vi "LuaPush.vi"(1 "Variant":variant, 2 "L In":u64, 3 "Lua Dll":path) -> (0 "L Out":u64)   [LabVIEW 2014]
uses:
  <vilib>/Utility/VariantDataType/Type.ctl
  <vilib>/Utility/VariantDataType/VariantType.lvlib
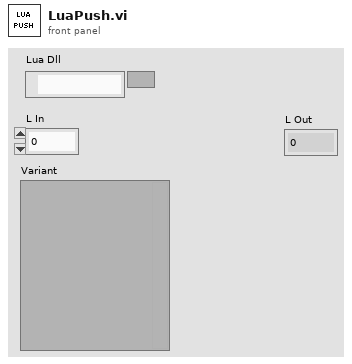
[diagram p1: front panel]
types:
  T1 = typedef "VariantType.lvlib/Type.ctl" = enum8{"Invalid Type", "Void", "I8", "I16", "I32", "I64", "U8", "U16", "U32", "U64", "Single Float", "Double Float", "Extended Float", "Single Complex", "Double Complex", "Extended Complex", "Enum U8", "Enum U16", "Enum U32", "Enum U64", "Single Float With Unit", "Double Float With Unit", "Extended Float With Unit", "Single Complex with Unit", "Double Complex with Unit", "Extended Complex with Unit", "Boolean", "String", "Path", "Picture", "Tag", "Array", "Cluster", "Variant", "LV Variant", "Waveform", "Timestamp", "Digital Waveform", "Digital Data", "ExpressData", "Refnum", "External Data", "VI", "Poly VI", "LabVIEW Class Instance", "Fixed Point"}
  T2 = typedef "VariantType.lvlib/RefnumType.ctl" = enum16{"NotARefnum", "UnknownRefnum", "Generic", "Datalog", "ByteStream", "Device", "Occurence", "TCPNetConnection", "Auto", "Menu", "Imaq", "Hardware", "DataSocket", "Visa", "IVI", "UDPNetConnection", "Notifier", "Queue", "Irda", "EventReg", "DotNet", "UserEvent", "Callback", "UNUSED_EMPTY_POSITION", "BlueToothNetConnection", "LVObjApp", "LVObjVI", "LVObjUnknown", "GenericClass", "UserDefinedRefnumTag", "DataValue", "RT FIFO", "TDMS File"}
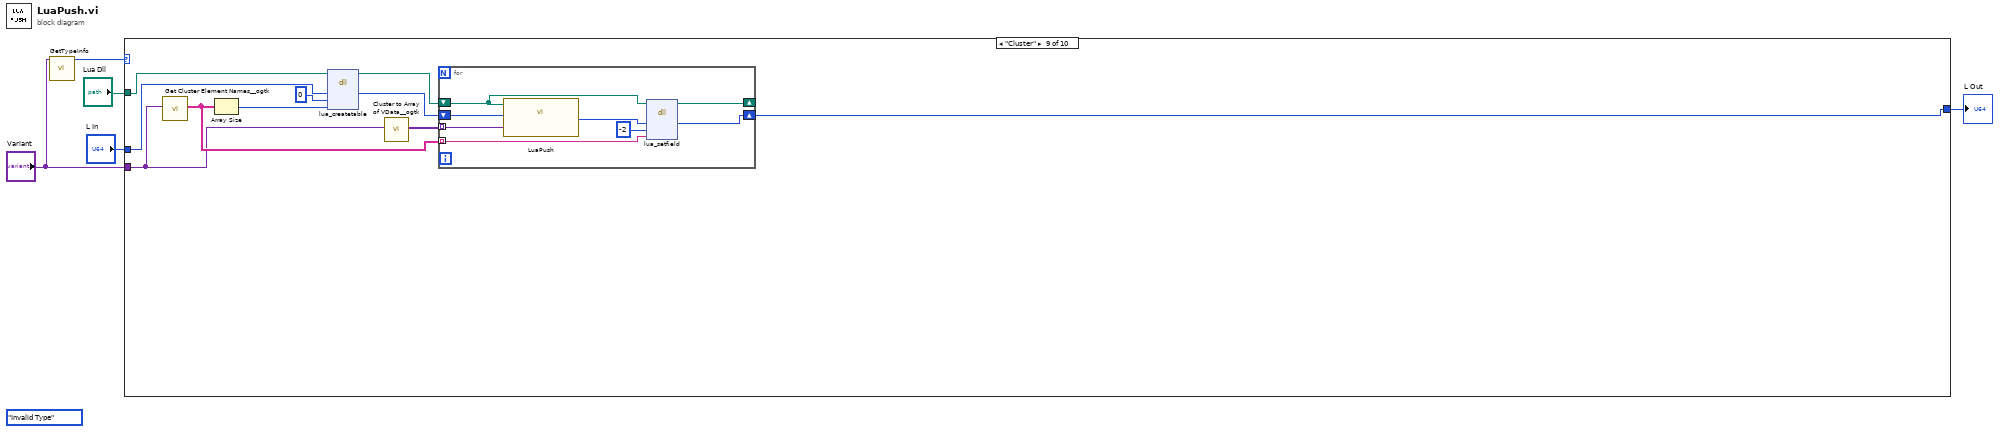
[diagram p0: block diagram]
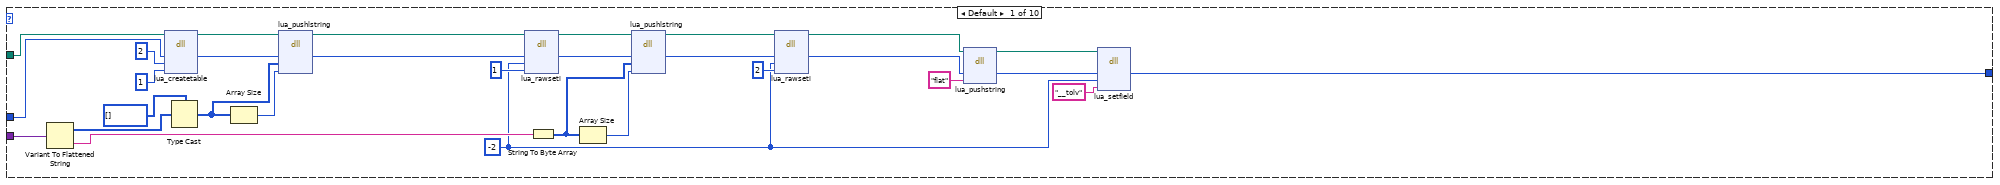
[diagram p2: hidden frame]
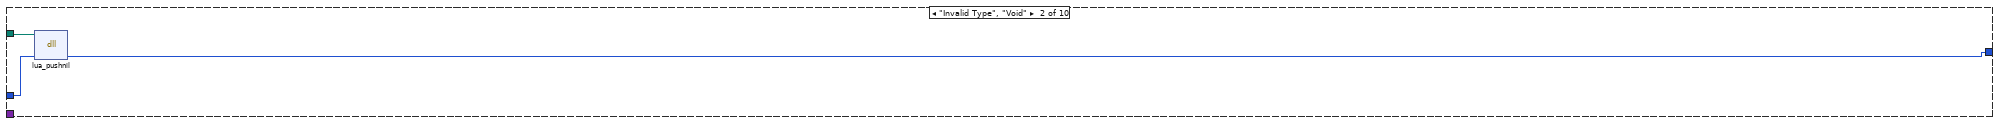
[diagram p3: hidden frame]
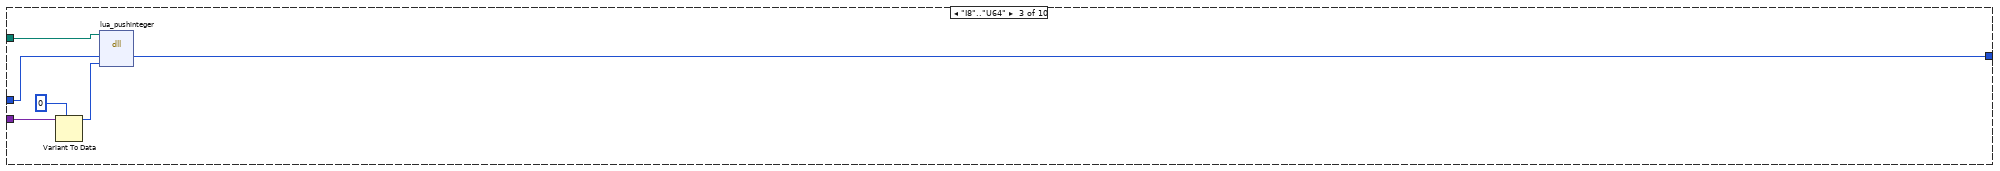
[diagram p4: hidden frame]
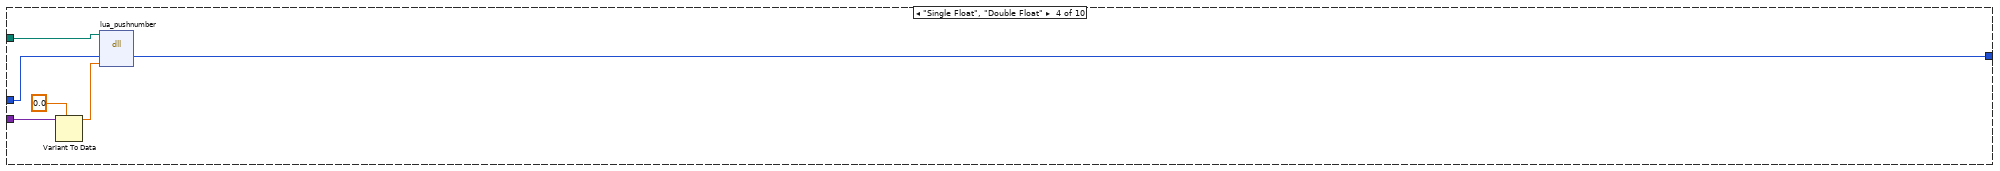
[diagram p5: hidden frame]
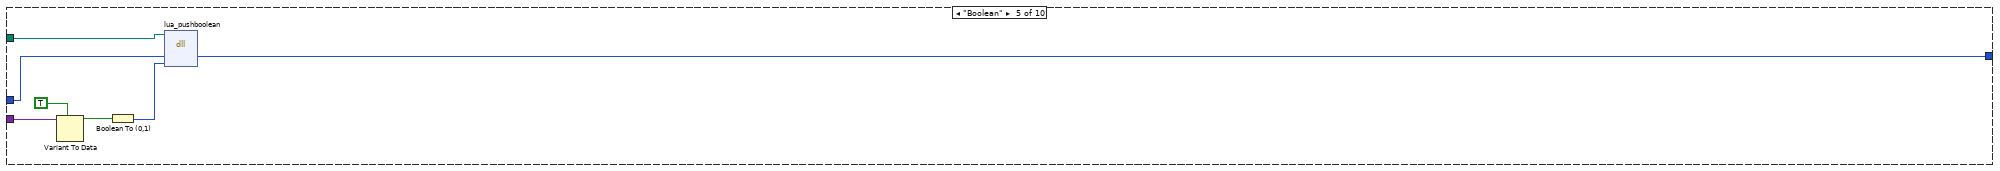
[diagram p6: hidden frame]
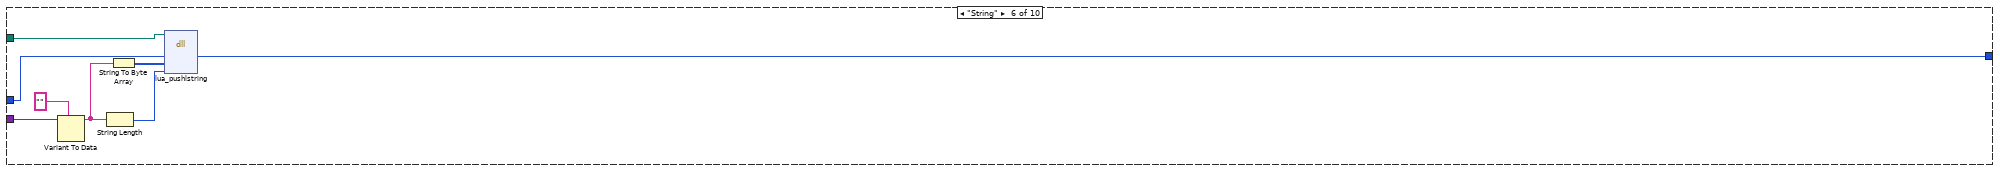
[diagram p7: hidden frame]
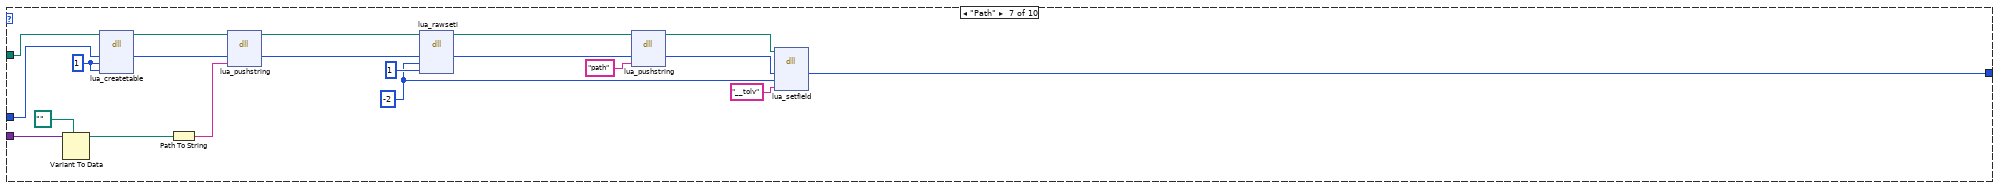
[diagram p8: hidden frame]
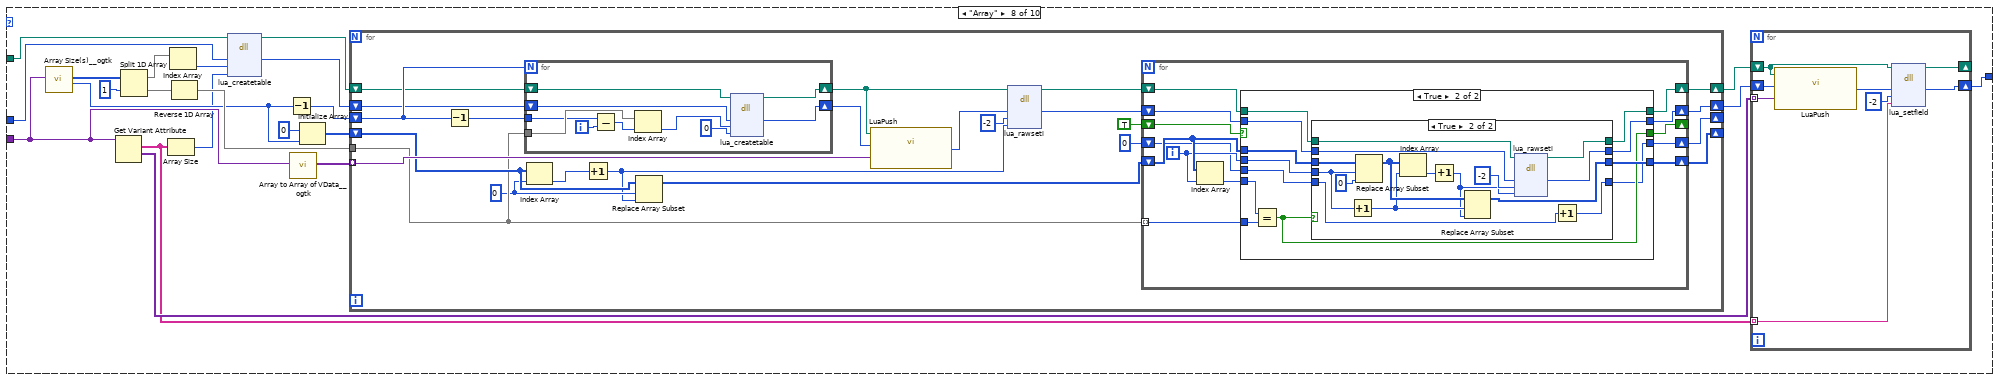
[diagram p9: hidden frame]
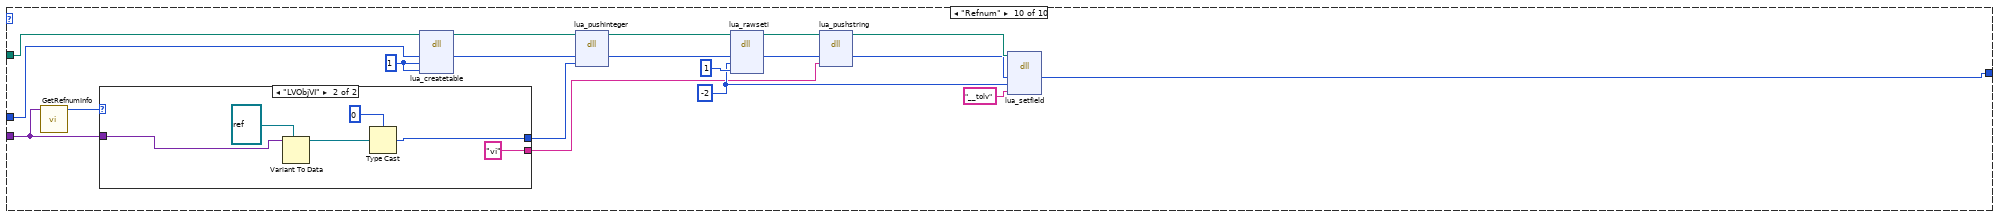
[diagram p12: hidden frame]
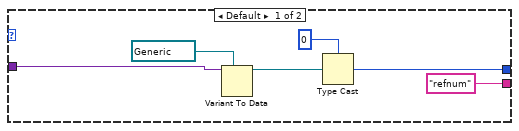
[diagram p13: hidden frame]
diagram:
  (unwired) Type."Invalid Type" ("Type Enum")
  n1 = call <vilib>:"GetTypeInfo.vi"("Variant"="Variant") -> ("Type Enum"=w5:T1)  [unwired: 6 in, 4 out]
  n2 = case shown="\"Cluster\"" w5 {
    tunnel: "Lua Dll" -> [w35 w38 w41 w47 w56 w64 w77 w95 w206 w221]
    tunnel: "L In" -> [w34 w37 w40 w46 w55 w63 w76 w93 w207 w219]
    tunnel: "Variant" -> [w26 _ w44 w50 w57 w65 w71 w99 w199 w223]
    tunnel: [w6 w36 w39 w45 w51 w58 w66 w86 w201 w216] -> w1
    frame Default {
      w7 = -2 ("n")
      n3 = Variant To Flattened String(Variant=w26) -> (data string=w19:string, 1:w25:i16[])
      n4 = dll-call lib="lua5.dll" fn="lua_createtable"(path in=w35, "L"=w34, "narr"=2, "nrec"=1) -> (path out=w22:path, "L"=w23:u64)  [unwired: 5 in, 1 out]
      n5 = Type Cast(type=u8[] [], x=w25) -> (*(type *) &x=w10:u8[])
      n6 = Array Size(array=w10) -> (size(s)=w9:i32)
      n7 = dll-call lib="lua5.dll" fn="lua_pushlstring"(path in=w22, "L"=w23, "str"=w10, "len"=w9) -> (path out=w21:path, "L"=w20:u64)  [unwired: 5 in, 1 out]
      n8 = dll-call lib="lua5.dll" fn="lua_rawseti"(path in=w21, "L"=w20, "n"=w7, "i"=1) -> (path out=w18:path, "L"=w15:u64)  [unwired: 5 in, 1 out]
      n9 = String To Byte Array(string=w19) -> (unsigned byte array=w12:u8[])
      n10 = Array Size(array=w12) -> (size(s)=w11:i32)
      n11 = dll-call lib="lua5.dll" fn="lua_pushlstring"(path in=w18, "L"=w15, "str"=w12, "len"=w11) -> (path out=w17:path, "L"=w14:u64)  [unwired: 5 in, 1 out]
      n12 = dll-call lib="lua5.dll" fn="lua_rawseti"(path in=w17, "L"=w14, "n"=w7, "i"=2) -> (path out=w16:path, "L"=w13:u64)  [unwired: 5 in, 1 out]
      n13 = dll-call lib="lua5.dll" fn="lua_pushstring"(path in=w16, "L"=w13, "str"="flat") -> (path out=w31:path, "L"=w30:u64)  [unwired: 4 in, 1 out]
      n14 = dll-call lib="lua5.dll" fn="lua_setfield"(path in=w31, "L"=w30, "n"=w7, "i"="__tolv") -> ("L"=w6:u64)  [unwired: 5 in, 2 out]
    }
    frame "Invalid Type", "Void" {
      n15 = dll-call lib="lua5.dll" fn="lua_pushnil"(path in=w38, "L"=w37) -> ("L"=w36:u64)  [unwired: 3 in, 2 out]
    }
    frame "I8".."U64" {
      n16 = Variant To Data(type=i64 0 ("n"), Variant=w44) -> (data=w42:i64)  [unwired: 1 in, 1 out]
      n17 = dll-call lib="lua5.dll" fn="lua_pushinteger"(path in=w41, "L"=w40, "n"=w42) -> ("L"=w39:u64)  [unwired: 4 in, 2 out]
    }
    frame "Single Float", "Double Float" {
      n18 = Variant To Data(type=0.0 ("n"), Variant=w50) -> (data=w48:dbl)  [unwired: 1 in, 1 out]
      n19 = dll-call lib="lua5.dll" fn="lua_pushnumber"(path in=w47, "L"=w46, "n"=w48) -> ("L"=w45:u64)  [unwired: 4 in, 2 out]
    }
    frame "Boolean" {
      n20 = Variant To Data(type=TRUE, Variant=w57) -> (data=w53:bool)  [unwired: 1 in, 1 out]
      n21 = Boolean To (0,1)(Boolean=w53) -> (0, 1=w52:i16)
      n22 = dll-call lib="lua5.dll" fn="lua_pushboolean"(path in=w56, "L"=w55, "n"=w52) -> ("L"=w51:u64)  [unwired: 4 in, 2 out]
    }
    frame "String" {
      n23 = Variant To Data(type="", Variant=w65) -> (data=w60:string)  [unwired: 1 in, 1 out]
      n24 = String Length(string=w60) -> (length=w61:i32)
      n25 = String To Byte Array(string=w60) -> (unsigned byte array=w59:u8[])
      n26 = dll-call lib="lua5.dll" fn="lua_pushlstring"(path in=w64, "L"=w63, "str"=w59, "len"=w61) -> ("L"=w58:u64)  [unwired: 5 in, 2 out]
    }
    frame "Path" {
      w78 = 1 ("narr")
      w79 = -2 ("n")
      n27 = Variant To Data(type=path "" ("path"), Variant=w71) -> (data=w69:path)  [unwired: 1 in, 1 out]
      n28 = dll-call lib="lua5.dll" fn="lua_createtable"(path in=w77, "L"=w76, "narr"=w78, "nrec"=w78) -> (path out=w75:path, "L"=w73:u64)  [unwired: 5 in, 1 out]
      n29 = Path To String(path=w69) -> (string=w68:string)
      n30 = dll-call lib="lua5.dll" fn="lua_pushstring"(path in=w75, "L"=w73, "str"=w68) -> (path out=w74:path, "L"=w72:u64)  [unwired: 4 in, 1 out]
      n31 = dll-call lib="lua5.dll" fn="lua_rawseti"(path in=w74, "L"=w72, "n"=w79, "i"=1) -> (path out=w82:path, "L"=w81:u64)  [unwired: 5 in, 1 out]
      n32 = dll-call lib="lua5.dll" fn="lua_pushstring"(path in=w82, "L"=w81, "str"="path") -> (path out=w85:path, "L"=w84:u64)  [unwired: 4 in, 1 out]
      n33 = dll-call lib="lua5.dll" fn="lua_setfield"(path in=w85, "L"=w84, "n"=w79, "i"="__tolv") -> ("L"=w66:u64)  [unwired: 5 in, 2 out]
    }
    frame "Array" {
      n34 = call <userlib>:"Array Size(s)__ogtk.vi"("Array"=w99) -> ("N dims"=w100:u32, "Size(s)"=w101:u32[])  [unwired: 8 in, 1 out]
      n35 = Get Variant Attribute(Variant=w99) -> (names=w97:string[], values=w98:variant[])  [unwired: 3 in, 2 out]
      n36 = Split 1D Array(array=w101, index=1) -> (first subarray=w88:u32[], second subarray=w103:u32[])
      n37 = Array Size(array=w97) -> (size(s)=w96:i32)
      n38 = Index Array(array=w88) -> (element=w87:u32)  [unwired: 1 in]
      n39 = Reverse 1D Array(array=w103) -> (reversed array=w104:u32[])
      n40 = dll-call lib="lua5.dll" fn="lua_createtable"(path in=w95, "L"=w93, "narr"=w87, "nrec"=w96) -> (path out=w94:path, "L"=w92:u64)  [unwired: 5 in, 1 out]
      n41 = Decrement(x=w100) -> (x-1=w89:u32)
      n42 = call <userlib>:"Array to Array of VData__ogtk.vi"("MultiD Array"=w99) -> ("1D Array of Variants"=w107:variant[])  [unwired: 9 in, 1 out]
      n43 = Initialize Array(0 ("nrec"), w100) -> (w105:i32[])
      n44 = for {
        tunnel: w107 -> [w136] mode=indexing
        shift-right: [w126] -> w91
        shift-left: w94 -> [w122]
        shift-right: [w125] -> w90
        shift-left: w92 -> [w121]
        shift-right: [w129] -> _
        shift-left: w105 -> [w133]
        tunnel: w104 -> [w128]
        shift-right: [w124] -> _
        shift-left: w89 -> [w123]
        w117 = 0 ("index")
        n45 = Decrement(x=w123) -> (x-1=w127:u32)
        n46 = for {
          N: w123 -> [_]
          shift-right: [w139] -> w137
          shift-left: w122 -> [w148]
          shift-right: [w146] -> w120
          shift-left: w121 -> [w147]
          tunnel: w128 -> [w144]
          tunnel: w127 -> [w140]
          i -> [w142]
          n47 = Subtract(x=w140, y=w142) -> (x-y=w141:u32)
          n48 = Index Array(array=w144, index=w141) -> (element=w143:u32)
          n49 = dll-call lib="lua5.dll" fn="lua_createtable"(path in=w148, "L"=w147, "narr"=w143, "nrec"=0) -> (path out=w139:path, "L"=w146:u64)  [unwired: 5 in, 1 out]
        }
        n50 = Index Array(array=w133, index=w117) -> (element=w118:i32)
        n51 = Increment(x=w118) -> (x+1=w116:i32)
        n52 = Replace Array Subset(array=w133, new element=w116, index=w117) -> (w132:i32[])
        n53 = call "LuaPush.vi"("Variant"=w136, "L In"=w120, "Lua Dll"=w137) -> ("L Out"=w135:u64)
        n54 = dll-call lib="lua5.dll" fn="lua_rawseti"(path in=w137, "L"=w135, "n"=-2, "i"=w116) -> (path out=w138:path, "L"=w134:u64)  [unwired: 5 in, 1 out]
        n55 = for {
          shift-right: [w153] -> w129
          shift-left: w132 -> [w157]
          tunnel: w128 -> [w159] mode=indexing
          shift-right: [w151] -> w125
          shift-left: w134 -> [w154]
          shift-right: [w152] -> w126
          shift-left: w138 -> [w155]
          shift-right: [w158] -> _
          shift-left: TRUE -> [w161]
          shift-right: [w149] -> w124
          shift-left: 0 ("new element/subarray") -> [w150]
          i -> [w156]
          n56 = Index Array(array=w157, index=w156) -> (element=w160:i32)
          n57 = case shown="True" w161 {
            selector: w161 -> [w166 _]
            tunnel: [w165 w178] -> w153
            tunnel: [w164 w177] -> w152
            tunnel: [w163 w176] -> w151
            tunnel: w160 -> [_ w175]
            tunnel: w159 -> [_ w174]
            tunnel: [w166 w173] -> w158
            tunnel: w157 -> [w165 w172]
            tunnel: w156 -> [_ w171]
            tunnel: w155 -> [w164 w170]
            tunnel: w154 -> [w163 w169]
            tunnel: w150 -> [w162 w168]
            tunnel: [w162 w167] -> w149
            frame False {
            }
            frame True {
              n58 = Equal?(x=w175, y=w174) -> (x = y?=w173:bool)
              n59 = case shown="True" w173 {
                tunnel: [w180 w189] -> w178
                tunnel: [w182 w194] -> w177
                tunnel: [w181 w193] -> w176
                tunnel: w172 -> [w180 w192]
                tunnel: w171 -> [_ w191]
                tunnel: w170 -> [w182 w186]
                tunnel: w169 -> [w181 w185]
                tunnel: w168 -> [w179 w184]
                tunnel: [w179 w183] -> w167
                frame False {
                }
                frame True {
                  n60 = Increment(x=w191) -> (x+1=w188:i32)
                  n61 = Replace Array Subset(array=w192, new element=0 ("new element/subarray"), index=w191) -> (w190:i32[])
                  n62 = Index Array(array=w190, index=w188) -> (element=w195:i32)
                  n63 = Increment(x=w195) -> (x+1=w187:i32)
                  n64 = Replace Array Subset(array=w190, new element=w187, index=w188) -> (w189:i32[])
                  n65 = dll-call lib="lua5.dll" fn="lua_rawseti"(path in=w186, "L"=w185, "n"=-2, "i"=w187) -> (path out=w194:path, "L"=w193:u64)  [unwired: 5 in, 1 out]
                  n66 = Increment(x=w184) -> (x+1=w183:i32)
                }
              }
            }
          }
        }
      }
      n67 = for {
        tunnel: w97 -> [w109] mode=indexing
        tunnel: w98 -> [w114] mode=indexing
        shift-right: [w111] -> _
        shift-left: w91 -> [w112]
        shift-right: [w110] -> w86
        shift-left: w90 -> [w115]
        n68 = call "LuaPush.vi"("Variant"=w114, "L In"=w115, "Lua Dll"=w112) -> ("L Out"=w113:u64)
        n69 = dll-call lib="lua5.dll" fn="lua_setfield"(path in=w112, "L"=w113, "n"=-2, "i"=w109) -> (path out=w111:path, "L"=w110:u64)  [unwired: 5 in, 1 out]
      }
    }
    frame "Cluster" {
      n70 = call <userlib>:"Get Cluster Element Names__ogtk.vi"("Cluster"=w199) -> ("Element Names"=w200:string[])  [unwired: 9 in, 1 out]
      n71 = Array Size(array=w200) -> (size(s)=w202:i32)
      n72 = dll-call lib="lua5.dll" fn="lua_createtable"(path in=w206, "L"=w207, "narr"=0, "nrec"=w202) -> (path out=w205:path, "L"=w204:u64)  [unwired: 5 in, 1 out]
      n73 = call <userlib>:"Cluster to Array of VData__ogtk.vi"("Cluster"=w199) -> ("Array of VData"=w198:variant[])  [unwired: 9 in, 1 out]
      n74 = for {
        tunnel: w200 -> [w209] mode=indexing
        shift-right: [w212] -> _
        shift-left: w205 -> [w213]
        shift-right: [w211] -> w201
        shift-left: w204 -> [w215]
        tunnel: w198 -> [w208] mode=indexing
        n75 = call "LuaPush.vi"("Variant"=w208, "L In"=w215, "Lua Dll"=w213) -> ("L Out"=w214:u64)
        n76 = dll-call lib="lua5.dll" fn="lua_setfield"(path in=w213, "L"=w214, "n"=-2, "i"=w209) -> (path out=w212:path, "L"=w211:u64)  [unwired: 5 in, 1 out]
      }
    }
    frame "Refnum" {
      w217 = 1 ("narr")
      w225 = -2 ("n")
      n77 = call <vilib>:"GetRefnumInfo.vi"("Variant"=w223) -> ("ReferenceType"=w234:T2)  [unwired: 7 in, 3 out]
      n78 = case shown="\"LVObjVI\"" w234 {
        tunnel: ["refnum" ("str") "vi" ("str")] -> w224
        tunnel: w223 -> [w239 w244]
        tunnel: [w235 w241] -> w222
        frame Default {
          n79 = Variant To Data(type=refnum<vi> refnum ("reference"), Variant=w239) -> (data=w237:refnum<vi>)  [unwired: 1 in, 1 out]
          n80 = Type Cast(type=u32 0 ("i"), x=w237) -> (*(type *) &x=w235:u32)
        }
        frame "LVObjVI" {
          n81 = Variant To Data(type=refnum<vi> refnum ("vi reference"), Variant=w244) -> (data=w243:refnum<vi>)  [unwired: 1 in, 1 out]
          n82 = Type Cast(type=u32 0 ("i"), x=w243) -> (*(type *) &x=w241:u32)
        }
      }
      n83 = dll-call lib="lua5.dll" fn="lua_createtable"(path in=w221, "L"=w219, "narr"=w217, "nrec"=w217) -> (path out=w220:path, "L"=w218:u64)  [unwired: 5 in, 1 out]
      n84 = dll-call lib="lua5.dll" fn="lua_pushinteger"(path in=w220, "L"=w218, "n"=w222) -> (path out=w230:path, "L"=w228:u64)  [unwired: 4 in, 1 out]
      n85 = dll-call lib="lua5.dll" fn="lua_rawseti"(path in=w230, "L"=w228, "n"=w225, "i"=1) -> (path out=w229:path, "L"=w227:u64)  [unwired: 5 in, 1 out]
      n86 = dll-call lib="lua5.dll" fn="lua_pushstring"(path in=w229, "L"=w227, "str"=w224) -> (path out=w233:path, "L"=w232:u64)  [unwired: 4 in, 1 out]
      n87 = dll-call lib="lua5.dll" fn="lua_setfield"(path in=w233, "L"=w232, "n"=w225, "i"="__tolv") -> ("L"=w216:u64)  [unwired: 5 in, 2 out]
    }
  }
  "L Out" <- w1
